vi "Process.vi"(8 "error in":errorcluster, 11 "Qbus in":refnum<class "Qbus.lvclass">) -> (0 "error out":errorcluster)   [LabVIEW 2021, in "AudioGenManageConnectionProcess.lvlib"]
uses:
  AudioGenManageConnectionProcess.lvlib
  <vilib>/addons/Qbus/Qbus.lvclass
  shared/logger process/controls/event.ctl
  <vilib>/NI/STM/TCP/Write Meta Data (TCP Ref).vi
  <vilib>/NI/STM/TCP/Get Connection Reference (TCP).vi
  <vilib>/NI/STM/TCP/Write Meta Data (TCP Clst).vi
  <vilib>/NI/STM/TCP/Write Message (TCP).vi
  <vilib>/NI/STM/Connection Manager/TCP/TCP Connection Manager.vi
  shared/logger process/EventLoggerProcess.lvlib
  <vilib>/NI/STM/NI STM.lvlib
  subVIs/utility/AudioGenUtility.lvlib
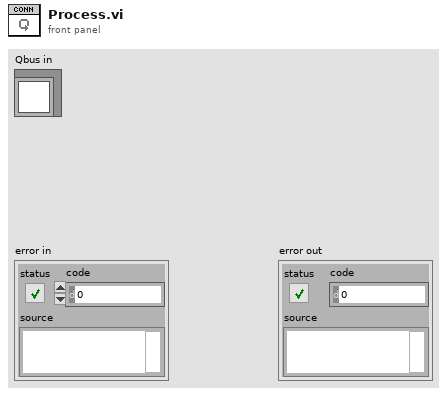
[diagram p1: front panel]
types:
  T1 = typedef "EventLoggerProcess.lvlib/event.ctl" = cluster{"name":string, "description":string}
  T2 = typedef "AudioGenTypeDefs.lvlib/service settings.ctl" = cluster{"port":u32, "enable debug log":bool}
  T3 = typedef "NI STM.lvlib/TCP Connection Info.ctl" = cluster{"connection ID":refnum<k5>, "meta data":T4[]}
  T4 = typedef "NI STM.lvlib/MetaDataElement.ctl" = string
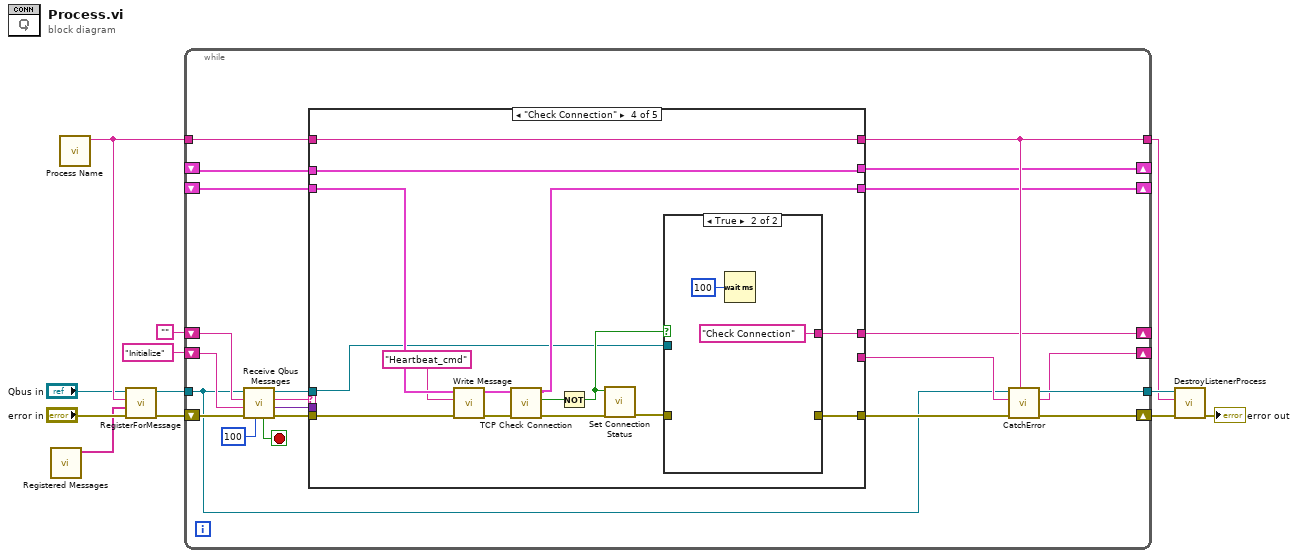
[diagram p0: block diagram]
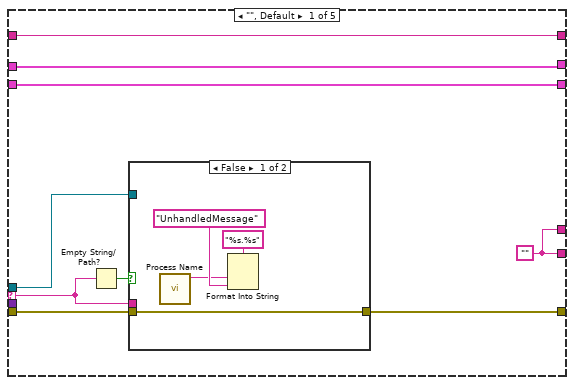
[diagram p2: hidden frame]
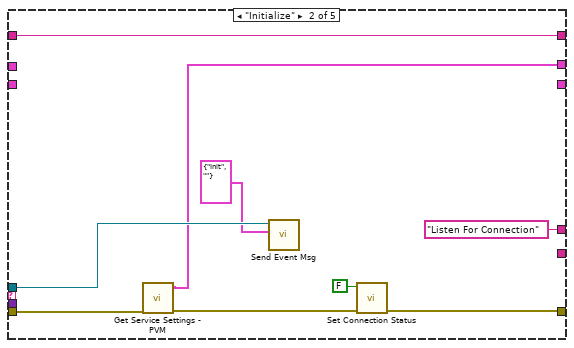
[diagram p4: hidden frame]
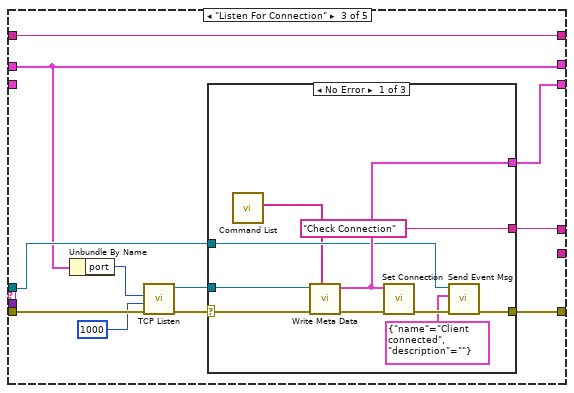
[diagram p5: hidden frame]
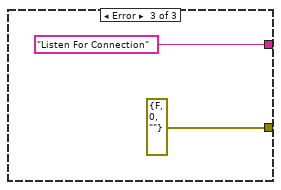
[diagram p7: hidden frame]
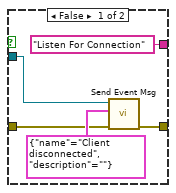
[diagram p8: hidden frame]
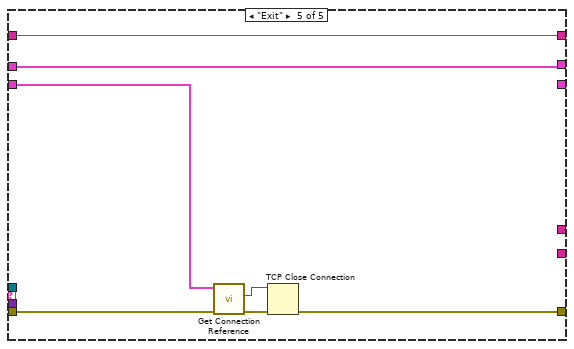
[diagram p9: hidden frame]
diagram:
  n1 = call "Registered Messages.vi"() -> ("registered messages"=w5:string[])  [unwired: 11 in]
  n2 = call "Process Name.vi"() -> ("process name"=w8:string)  [unwired: 11 in]
  n3 = call <vilib>:"RegisterForMessage.vi"("error in (no error)"="error in", "message names"=w5, "process name"=w8, "Qbus in"="Qbus in") -> ("error in (no error)"=w11:errorcluster, "Qbus out"=w12:refnum<class "Qbus.lvclass">)  [unwired: 6 in]
  n4 = while {
    shift-right: [w20] -> _
    shift-left: "" -> [w33]
    tunnel: w12 -> [w18]
    tunnel: w8 -> [w17]
    tunnel: [w27] -> w3
    tunnel: [w22] -> w1
    shift-right: [w26] -> _
    shift-left: "Initialize" -> [w29]
    shift-right: [w28] -> w4
    shift-left: w11 -> [w25]
    shift-right: [w16] -> _
    shift-left: _ -> [w15]
    shift-right: [w14] -> _
    shift-left: _ -> [w13]
    stop <- w34 stop-if-true
    n5 = call "Receive Qbus Messages.vi"("timeout(ms)"=100 ("milliseconds to wait"), "error in (no error)"=w25, "priority action"=w29, "default action"=w33, "Qbus in"=w18) -> ("error out"=w32:errorcluster, "message value"=w30:variant, "action"=w24:string, "Qbus out"=w31:refnum<class "Qbus.lvclass">, "exit"=w34:bool)  [unwired: 2 in]
    n6 = case shown="\"Check Connection\"" w24 {
      selector: w24 -> [w40 _ _ _ _]
      tunnel: w32 -> [w42 w51 w67 w95 w107]
      tunnel: w31 -> [w38 w56 w60 w83 _]
      tunnel: [w41 w53 w64 w90 w106] -> w19
      tunnel: w30 -> [_ _ _ _ _]
      tunnel: [w43 w57 w68 w96 w110] -> w22
      tunnel: w17 -> [w43 w57 w68 w96 w110]
      tunnel: [w37 _ _ _ _] -> w21
      tunnel: [w37 "Listen For Connection" w63 w89 _] -> w20
      tunnel: [w36 _ w61 w88 _] -> w16
      tunnel: w15 -> [w36 _ _ w94 w105]
      tunnel: [w35 w49 w59 w82 w104] -> w14
      tunnel: w13 -> [w35 _ w59 w82 w104]
      frame "", Default {
        w37 = ""
        n7 = Empty String/Path?(string/path=w40) -> (empty?=w39:bool)
        n8 = case shown="False" w39 {
          tunnel: [w44 w48] -> w41
          tunnel: w42 -> [w44 w48]
          tunnel: w40 -> [_ _]
          tunnel: w38 -> [_ _]
          frame False {
            n9 = call "Process Name.vi"() -> ("process name"=w45:string)  [unwired: 11 in]
            n10 = Format Into String(format string="%s.%s", w45, "UnhandledMessage" ("ProcessName")) -> ()  [unwired: 2 in, 2 out]
          }
          frame True {
          }
        }
      }
      frame "Initialize" {
        n11 = call "Get Service Settings - PVM.vi"("error in (no error)"=w51) -> ("error out"=w50:errorcluster, "service settings"=w49:T2)  [unwired: 9 in]
        n12 = call "Send Event Msg.vi"("event"=T1 {"name"="Init", "description"=""}, "Qbus in"=w56) -> ()  [unwired: 8 in, 2 out]
        n13 = call "Set Connection Status.vi"("error in (no error)"=w50, "connected"=FALSE) -> ("error out"=w53:errorcluster)  [unwired: 9 in]
      }
      frame "Listen For Connection" {
        n14 = Unbundle By Name(w59) -> ("port"=w58:u32)
        n15 = call <vilib>:"TCP Listen.vi"("error in (no error)"=w67, "timeout ms (wait forever: -1)"=1000, "port"=w58) -> ("error out"=w65:errorcluster, "connection ID"=w62:refnum<k5>)  [unwired: 1 in, 6 out]
        n16 = case shown="No Error" w65 {
          selector: w65 -> [w77 w79 _]
          tunnel: [w71 w79 errorcluster {"status"=FALSE, "code"=0, "source"=""} ("error IO")] -> w64
          tunnel: ["Check Connection" _ "Listen For Connection"] -> w63
          tunnel: w62 -> [w78 _ _]
          tunnel: [w74 _ _] -> w61
          tunnel: w60 -> [w72 _ _]
          frame No Error {
            n17 = call "Command List.vi"() -> ("TCP commands"=w69:string[])  [unwired: 11 in]
            n18 = call-poly <vilib>:"Write Meta Data.vi"("meta data"=w69, "error in"=w77, "connection ID"=w78) -> ("error out"=w75:errorcluster, "connection info out"=w74:T3)  [unwired: 2 in, 5 out]
            n19 = call "Set Connection.vi"("error in (no error)"=w75, "connection"=w74) -> ("error out"=w73:errorcluster)  [unwired: 9 in]
            n20 = call "Send Event Msg.vi"("error in"=w73, "event"=T1 {"name"="Client connected", "description"=""}, "Qbus in"=w72) -> ("error out"=w71:errorcluster)  [unwired: 7 in, 1 out]
          }
          frame Default {
          }
          frame Error {
          }
        }
      }
      frame "Check Connection" {
        n21 = call-poly <vilib>:"Write Message.vi"("error in"=w95, "name"="Heartbeat_cmd", "connection info in"=w94) -> ("error out"=w91:errorcluster, "connection info out"=w92:T3)  [unwired: 7 in]
        n22 = call <vilib>:"TCP Check Connection.vi"("error in"=w91, "connection in"=w92) -> ("error out"=w87:errorcluster, "disconnected?"=w85:bool, "connection out"=w88:T3)  [unwired: 7 in]
        n23 = Not(x=w85) -> (.not. x?=w84:bool)
        n24 = call "Set Connection Status.vi"("error in (no error)"=w87, "connected"=w84) -> ("error out"=w86:errorcluster)  [unwired: 9 in]
        n25 = case shown="True" w84 {
          tunnel: w86 -> [w99 _]
          tunnel: [w98 _] -> w90
          tunnel: ["Listen For Connection" "Check Connection"] -> w89
          tunnel: w83 -> [w97 _]
          frame False {
            n26 = call "Send Event Msg.vi"("error in"=w99, "event"=T1 {"name"="Client disconnected", "description"=""}, "Qbus in"=w97) -> ("error out"=w98:errorcluster)  [unwired: 7 in, 1 out]
          }
          frame True {
            n27 = Wait (ms)(milliseconds to wait=u32 100) -> ()  [unwired: 1 out]
          }
        }
      }
      frame "Exit" {
        n28 = call-poly <vilib>:"Get Connection Reference.vi"("error in"=w107, "connection info in"=w105) -> ("error out"=w108:errorcluster, "connection ID out"=w109:refnum<k5>)  [unwired: 8 out]
        n29 = TCP Close Connection(connection ID=w109, error in (no error)=w108) -> (error out=w106:errorcluster)  [unwired: 2 out]
      }
    }
    n30 = call <vilib>:"CatchError.vi"("source"=w22, "error in (no error)"=w19, "next action in"=w21, "Qbus in"=w18) -> ("error out"=w28:errorcluster, "next action out"=w26:string, "Qbus out"=w27:refnum<class "Qbus.lvclass">)  [unwired: 5 in]
  }
  n31 = call <vilib>:"DestroyListenerProcess.vi"("error in (no error)"=w4, "process name"=w1, "Qbus in"=w3) -> ("error in (no error)"=→"error out":errorcluster)  [unwired: 7 in, 1 out]
